vi "Serialize - Text.vi"(8 "(no error)":errorcluster, 11 "CRDS Cell Data in":refnum<class "CRDS Cell Data.lvclass">) -> (0 "error out":errorcluster, 2 "Serialized Text":string, 3 "CRDS Cell Data out":refnum<class "CRDS Cell Data.lvclass">)   [LabVIEW 2014, in "CRDS Lib.lvlib" / "CRDS Cell Data.lvclass"]
uses:
  CRDS Cell Data.lvclass
  CRDS Cell Data.lvclass/CRDS Cell Data.ctl
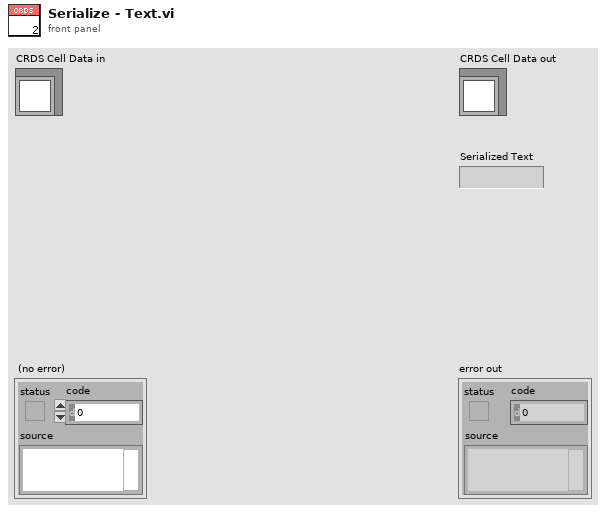
[diagram p1: front panel]
types:
  T1 = typedef "CRDS Lib.lvlib/extParam Ctl.ctl" = cluster{"Tau":sgl, "Tau0cor":sgl, "ext":sgl, "extCorr":sgl, "stdevTau":sgl, "eTau":sgl, "taucorr":sgl, "Tau0":sgl, "max":sgl}
  T2 = typedef "hkParam Ctl.ctl" = cluster{"rhDilFac":sgl, "Q":sgl, "Tmean":sgl, "extDilFac":sgl, "rhCell":sgl, "P":sgl, "T":sgl}
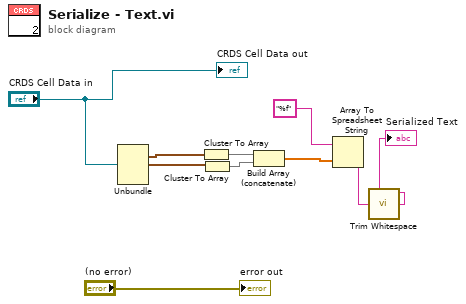
[diagram p0: block diagram]
diagram:
  n1 = Unbundle("CRDS Cell Data in") -> (w8:T1, w7:T2)  [unwired: 3 out]
  n2 = Cluster To Array(cluster=w8) -> (array=w6:sgl[])
  n3 = Cluster To Array(cluster=w7) -> (array=w5:sgl[])
  n4 = Build Array (concatenate)(w6, w5) -> (w4:sgl[])
  n5 = Array To Spreadsheet String(array=w4, 3:"%f" ("format string")) -> (spreadsheet string=w2:string)  [unwired: 1 in]
  n6 = call <vilib>:"Trim Whitespace.vi"("string"=w2) -> ("trimmed string"=→"Serialized Text":string)  [unwired: 1 in]
  "error out" <- "(no error)"
  "CRDS Cell Data out" <- "CRDS Cell Data in"
